vi "StateBallHandling.vi"(1 "Master State":T1(ring)) -> ()   [LabVIEW 2019]
doc: "This VI makes all decisions related to the ball handling subsystems including the intake, hopper, and magazine."
uses:
  dscommands.vi
  outputs.vi
panel:
  out "Time (ms)":u32
  in  "Magazine_Reverse_Power":dbl=-0.7 format="%#_13g"
  in  "Intake Speed":dbl=0.9
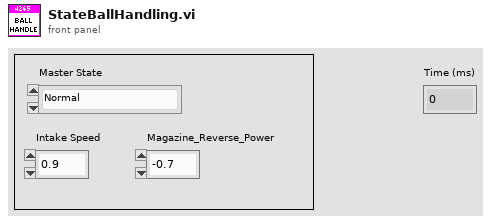
[diagram p1: front panel]
types:
  T1 = enum16{"Normal", "Control Rotation", "Control Position", "Climb"}
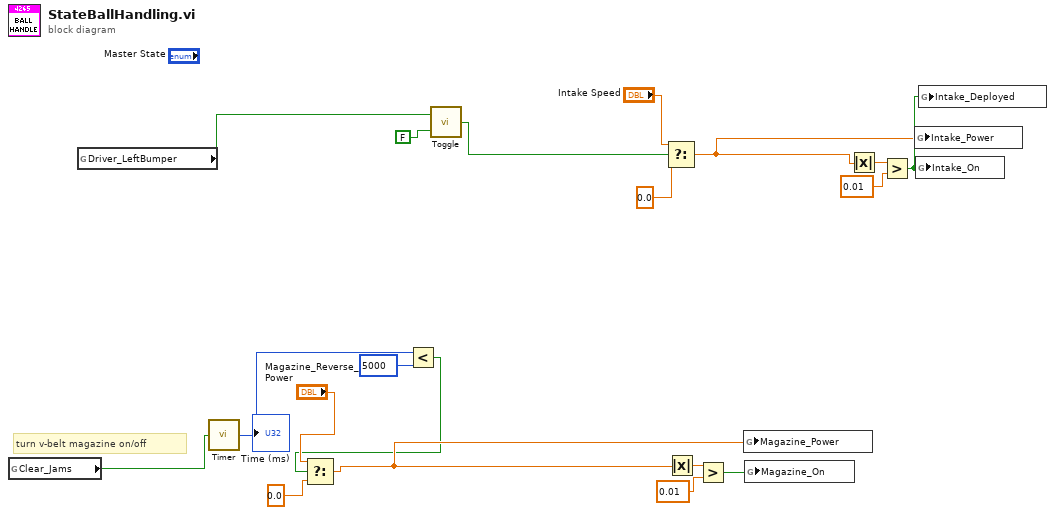
[diagram p0: block diagram]
diagram:
  # "turn v-belt magazine on/off"
  n1 = global read "dscommands.vi" "Clear_Jams"() -> (w4:bool)
  n2 = global read "dscommands.vi" "Driver_LeftBumper"() -> (w9:bool)
  n3 = call "Timer.vi"("Reset Timer"=w4) -> ("Time (ms)"=w3:u32)
  "Time (ms)" <- w3
  n4 = Less?(x=w3, y=5000) -> (x < y?=w1:bool)
  n5 = Select(t="Magazine_Reverse_Power", s=w1, f=0.0) -> (s? t:f=w5:dbl)
  n6 = call "Toggle.vi"("Initial State"=FALSE ("New State"), "Trigger"=w9) -> ("New State"=w10:bool)
  n7 = Select(t="Intake Speed", s=w10, f=0.0) -> (s? t:f=w11:dbl)
  n8 = Absolute Value(x=w5) -> (abs(x)=w17:dbl)
  n9 = Greater?(x=w17, y=0.01) -> (0:w15:bool)
  n10 = global write "outputs.vi" "Magazine_Power"(w5) -> ()
  n11 = global write "outputs.vi" "Magazine_On"(w15) -> ()
  n12 = Absolute Value(x=w11) -> (abs(x)=w19:dbl)
  n13 = Greater?(x=w19, y=0.01) -> (0:w14:bool)
  n14 = global write "outputs.vi" "Intake_Power"(w11) -> ()
  n15 = global write "outputs.vi" "Intake_On"(w14) -> ()
  n16 = global write "outputs.vi" "Intake_Deployed"(w14) -> ()
